vi "FTW-Container-Probe.vi"(11 "FTW-Container In":refnum<class "FTW-Container.lvclass">) -> (2 "Value String":string, 3 "Boolean":bool)   [LabVIEW 2015, in "FTW-Container.lvclass"]
uses:
  FTW-Container.lvclass
panel:
  out "JSON String":string
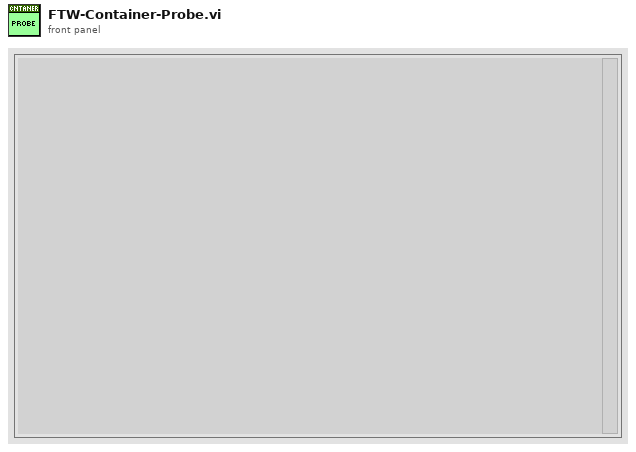
[diagram p1: front panel]
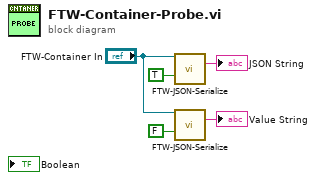
[diagram p0: block diagram]
diagram:
  n1 = call "FTW-JSON-Serialize.vi"("JSON"="FTW-Container In", "Pretty Print"=TRUE) -> ("JSON String (UTF-8)"=→"JSON String":string)  [unwired: 11 in, 2 out]
  n2 = call "FTW-JSON-Serialize.vi"("JSON"="FTW-Container In", "Pretty Print"=FALSE) -> ("JSON String (UTF-8)"=→"Value String":string)  [unwired: 11 in, 2 out]
